vi "Add Graphic Object.vi"(8 "error in (no error)":errorcluster, 10 "Graphic":refnum<class "Graphic.lvclass">, 11 "Canvas in":refnum<class "Canvas.lvclass">) -> (0 "error out":errorcluster, 2 "Graphic out":refnum<class "Graphic.lvclass">, 3 "Canvas out":refnum<class "Canvas.lvclass">)   [LabVIEW 2015, in "Canvas.lvclass"]
uses:
  Canvas.lvclass
  Graphic/Graphic.lvclass
  Canvas.lvclass/Canvas.ctl
  Graphic/Graphic.lvclass/Graphic.ctl
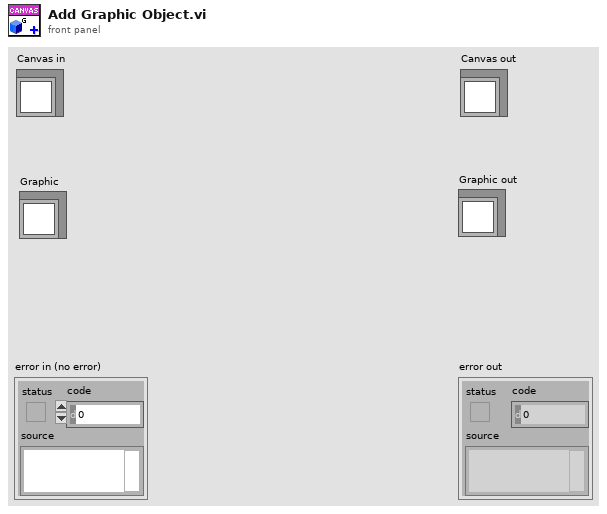
[diagram p1: front panel]
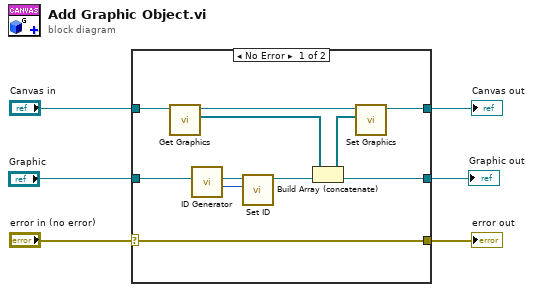
[diagram p0: block diagram]
diagram:
  n1 = case shown="No Error" "error in (no error)" {
    selector: "error in (no error)" -> [w14 w18]
    tunnel: [w14 w18] -> w5
    tunnel: [w11 w17] -> w3
    tunnel: "Canvas in" -> [w15 w17]
    tunnel: "Graphic" -> [w9 w16]
    tunnel: [w7 w16] -> w1
    frame No Error {
      n2 = call "Get Graphics.vi"("Canvas in"=w15) -> ("Graphics"=w12:refnum<class "Graphic.lvclass">[], "Canvas out"=w13:refnum<class "Canvas.lvclass">)  [unwired: 8 in, 1 out]
      n3 = call "ID Generator.vi"() -> ("ID"=w8:i32)  [unwired: 11 in]
      n4 = call "Set ID.vi"("ID"=w8, "Graphic in"=w9) -> ("Graphic out"=w7:refnum<class "Graphic.lvclass">)  [unwired: 8 in, 1 out]
      n5 = Build Array (concatenate)(w12, w7) -> (w10:refnum<class "Graphic.lvclass">[])
      n6 = call "Set Graphics.vi"("Graphics"=w10, "Canvas in"=w13) -> ("Canvas out"=w11:refnum<class "Canvas.lvclass">)  [unwired: 8 in, 1 out]
    }
    frame Error {
    }
  }
  "error out" <- w5
  "Canvas out" <- w3
  "Graphic out" <- w1
